vi "DAC Configure.vi"(8 "error in":errorcluster, 11 "DAC CS Humid in":refnum<class "DAC CS Humid.lvclass">) -> (0 "error out":errorcluster, 3 "DAC CS Humid out":refnum<class "DAC CS Humid.lvclass">)   [LabVIEW 2019, in "DAC.lvlib" / "DAC CS Humid.lvclass"]
uses:
  DAC CS Humid.lvclass
  C:/Users/wg/Documents/LV_Projects/test-stand/App/DAC/DAC.lvclass
  DAC.lvclass/DAC.ctl
  DAC CS Humid.lvclass/DAC CS Humid.ctl
  DAC.lvclass
  <vilib>/DAQmx/create/channels.llb/DAQmx Create Channel (AI-Current-Basic).vi
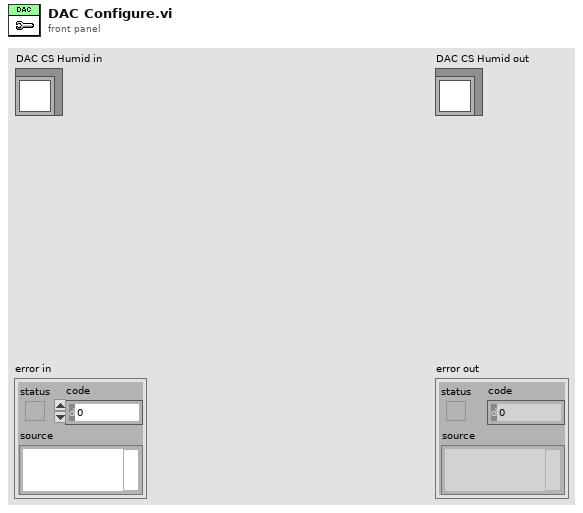
[diagram p1: front panel]
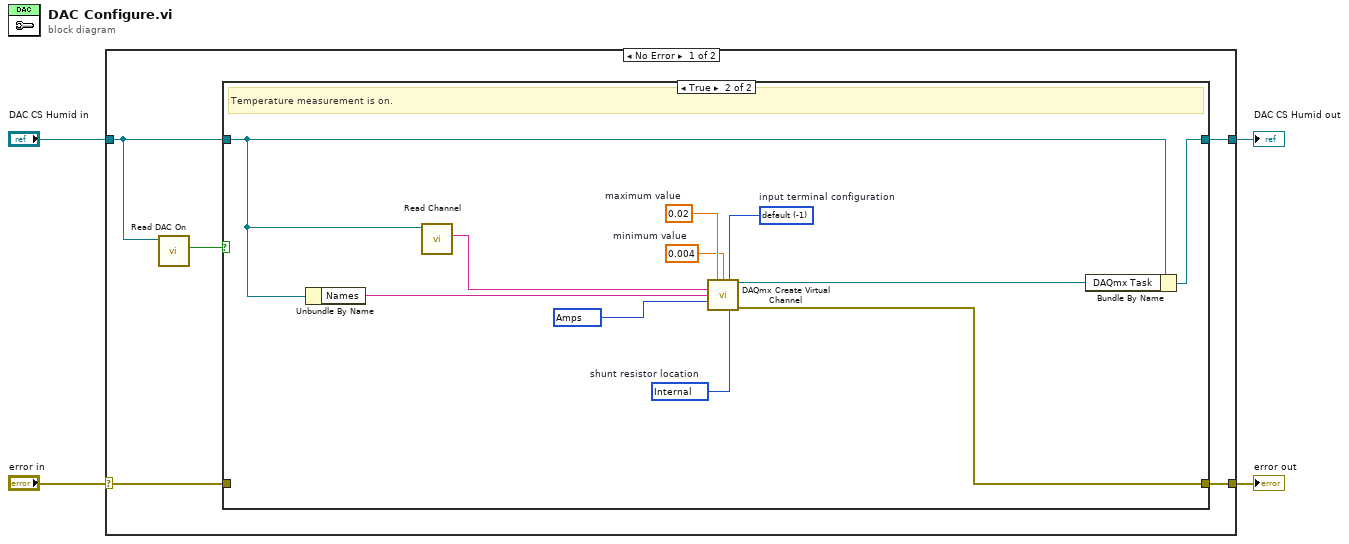
[diagram p0: block diagram]
diagram:
  n1 = case shown="No Error" "error in" {
    selector: "error in" -> [w6 w24]
    tunnel: [w5 w24] -> w4
    tunnel: [w7 w23] -> w3
    tunnel: "DAC CS Humid in" -> [w9 w23]
    frame No Error {
      n2 = call "Read DAC On.vi"("DAC in"=w9) -> ("DAC On"=w8:bool)  [unwired: 8 in, 2 out]
      n3 = case shown="True" w8 {
        tunnel: w9 -> [w11 w20]
        tunnel: [w11 w22] -> w7
        tunnel: w6 -> [w10 _]
        tunnel: [w10 w17] -> w5
        frame False {
          # "Temperature measurement is off."
        }
        frame True {
          w12 = 10200 items=["default"=-1, "Internal"=10200, "External"=10167]  # shunt resistor location
          w13 = -1 items=["default"=-1, "RSE"=10083, "NRSE"=10078, "Differential"=10106, "Pseudodifferential"=12529]  # input terminal configuration
          w14 = 10342 items=["Amps"=10342, "From Custom Scale"=10065] ("units")
          w15 = 0.004  # minimum value
          w16 = 0.02  # maximum value
          # "Temperature measurement is on."
          n4 = Unbundle By Name(w20) -> ("Names"=w21:string)
          n5 = call "Read Channel.vi"("DAC in"=w20) -> ("Channel"=w19:string)  [unwired: 8 in, 2 out]
          n6 = call-poly <vilib>:"DAQmx Create Virtual Channel.vi"("maximum value"=w16, "minimum value"=w15, "input terminal configuration"=w13, "physical channels"=w19, "name to assign"=w21, "units"=w14, "shunt resistor location"=w12) -> ("task out"=w18:refnum<k21>, "error out"=w17:errorcluster)  [unwired: 7 in]
          n7 = Bundle By Name(cluster=w20, "DAQmx Task"=w18) -> (w22:refnum<class "DAC CS Humid.lvclass">)
        }
      }
    }
    frame Error {
    }
  }
  "error out" <- w4
  "DAC CS Humid out" <- w3
